vi "PH_Sequencer_Watch.ProcEvents.vi"(0 "i ref in":refnum<vi>, 5 "error in (no error)":errorcluster) -> (14 "i ref out":refnum<vi>, 19 "error out":errorcluster)   [LabVIEW 2014, in "PH_Sequencer_Watch.lvlib"]
doc: "This method is used to define the events the object will listen to. Add your own events here."
uses:
  PH_Sequencer_Watch.lvlib
  PH_Beckhoff_PP_PU/PH_Beckhoff_PP_PU.HV Meas Tags.ctl
  PH_PP_Common/PH_PP_Common.PSU Tags.ctl
  PH_Common/DIM/PH_DIM.Event Declarer.ctl
  PH_PowerUnit_BaseClass/PH_PowerUnit_BaseClass.PP PU Tags.ctl
  CSCore/BaseProcess/BaseProcess.lvlib
  PH_Common/PH_Common.lvlib
  PH_Beckhoff_PP_PU/PH_Beckhoff_PP_PU.lvlib
  PH_PowerUnit_BaseClass/PH_PowerUnit_BaseClass.lvlib
  PH_PP_Common/PH_PP_Common.lvlib
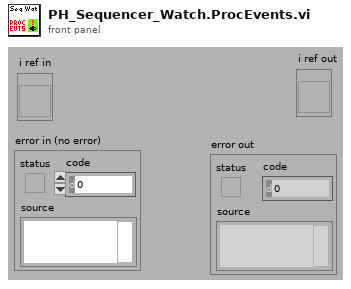
[diagram p1: front panel]
types:
  T1 = typedef "PH_PP_Common.lvlib/PH_PP_Common.PSU Tags.ctl" = enum16{"voltage-indicator", "peak-detect", "current", "voltage", "inihibit-indicator", "end-of-charge", "HV-on-indicator", "overtemperature", "interlock-indicator", "load-fault", "sum-fault", "HV-off-indicator", "DC-ok", "inhibit", "HV-on", "interlock", "reset", "Status", "Limits"}
  T2 = typedef "PH_Beckhoff_PP_PU.lvlib/PH_Beckhoff_PP_PU.HV Meas Tags.ctl" = enum16{"voltage-raw", "voltage"}
  T3 = typedef "PH_Common.lvlib/PH_DIM.Event Declarer.ctl" = cluster{"Service Name":string, "Selector":string}
  T4 = typedef "PH_PowerUnit_BaseClass.lvlib/PH_PowerUnit_BaseClass.PP PU Tags.ctl" = enum16{"Waiting-Time", "PU-in-Use"}
  T5 = typedef "PH_Sequencer_Watch.lvlib/PH_Sequencer_Watch.i attribute.ctl" = cluster{"GUI Refs":cluster{"Shot ID":refnum<vi>, "Sequencer SM State":refnum<vi>, "Remaining Time":refnum<vi>, "PHELIX_Timing_T2":refnum<vi>, "T2-Unit-Dummy":refnum<vi>, "fs_Synchrolock_Watch":refnum<vi>, "Experiment_Vacuum_Control_Experiment":refnum<vi>}, "Status Synchrolock":T6, "Exp - Pressure":dbl, "Exp - Limit":dbl, "Heads":T7[], "Refs BooleanState":refnum<vi>[]}
  T6 = typedef "PH_StatusHandler.lvlib/PH_StatusHandler.Status.ctl" = i16
  T7 = typedef "PH_Sequencer_Watch.lvlib/PH_Sequencer_Watch.Head Information.ctl" = cluster{"Ref Volt":refnum<vi>, "PU":T8}
  T8 = typedef "PH_PP_Common.lvlib/PH_PP_Common.PUs.ctl" = enum16{"no Info", "PA-19mm-1", "PA-19mm-2", "PA-45mm-PILC", "PA-45mm-MAIN", "MA-PU-1", "MA-PU-2", "MA-PU-3", "MA-PU-4", "MA-PU-5", "MA-PU-6", "MA-FR", "MA-PILC", "PA-45mm-DP"}
  T9 = typedef "PH_PP_Common.lvlib/PH_PP_Common.PSU Type.ctl" = enum16{"none", "Maxwell Standard", "DEL", "Maxwell ALE", "Continuum 601k"}
  T10 = typedef "BaseProcess.lvlib/BaseProcess.event definition.ctl" = cluster{"CAEEvtDef":T11, "Data Descriptor":T12}
  T11 = typedef "CAEObj.lvlib/CAEObj.event definition.ctl" = cluster{"URL":string, "enable":bool, "ignoreResID":bool}
  T12 = typedef "BaseProcess.lvlib/BaseProcess.descriptor string definition.ctl" = string
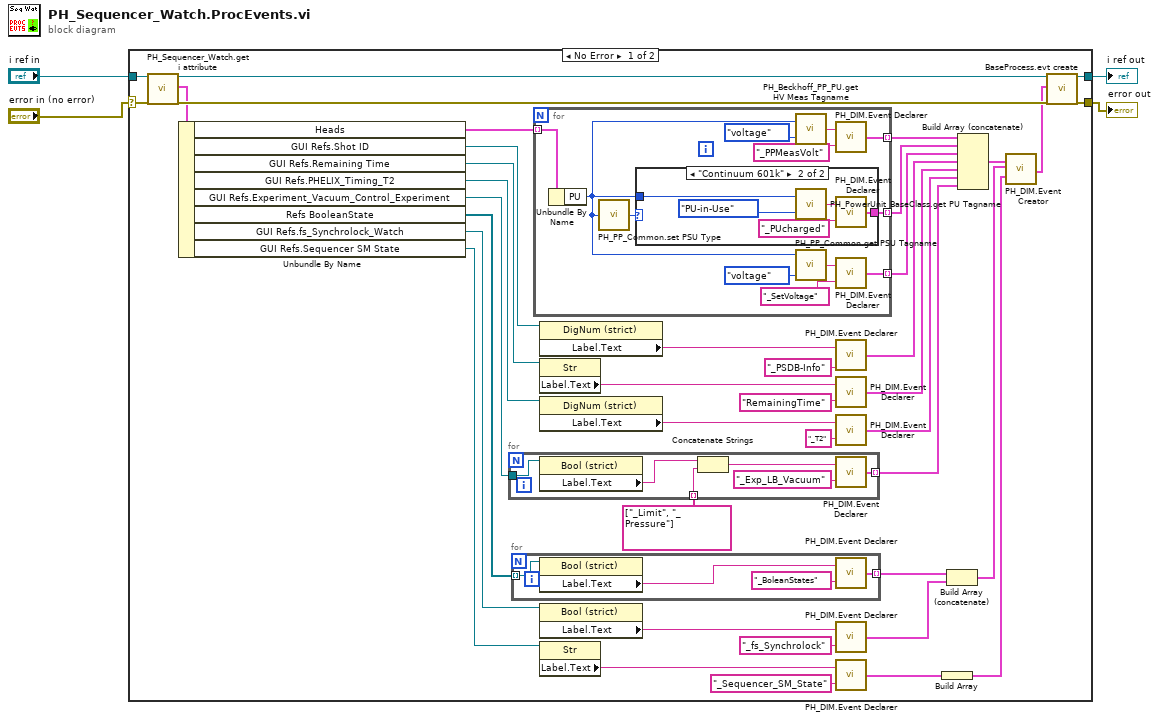
[diagram p0: block diagram]
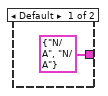
[diagram p2: hidden frame]
diagram:
  n1 = case shown="No Error" "error in (no error)" {
    selector: "error in (no error)" -> [w39 w73]
    tunnel: "i ref in" -> [w42 w74]
    tunnel: [w41 w74] -> w3
    tunnel: [w40 w73] -> w2
    frame No Error {
      n2 = call "PH_Sequencer_Watch.get i attribute.vi"("i ref in"=w42, "error in (no error)"=w39) -> ("i ref out"=w44:refnum<vi>, "i attribute"=w36:T5, "error out"=w43:errorcluster)  [unwired: 15 in]
      n3 = Unbundle By Name(w36) -> ("Heads"=w25:T7[], "GUI Refs.Shot ID"=w30:refnum<vi>, "GUI Refs.Remaining Time"=w32:refnum<vi>, "GUI Refs.PHELIX_Timing_T2"=w20:refnum<vi>, "GUI Refs.Experiment_Vacuum_Control_Experiment"=w10:refnum<vi>, "Refs BooleanState"=w17:refnum<vi>[], "GUI Refs.fs_Synchrolock_Watch"=w14:refnum<vi>, "GUI Refs.Sequencer SM State"=w7:refnum<vi>)
      n4 = for {
        tunnel: [w49] -> w8 mode=indexing
        tunnel: w10 -> [w47]
        tunnel: string[] ["_Limit", "_Pressure"] -> [w45] mode=indexing
        n5 = property class="Bool (strict)"(reference=w47) -> ("Label.Text"=w48:string)  [unwired: 1 in, 2 out]
        n6 = Concatenate Strings(w48, w45) -> (w46:string)
        n7 = call "PH_DIM.Event Declarer.vi"("Selector"="_Exp_LB_Vacuum" ("URL"), "Service Name"=w46) -> ("declared DIM Event"=w49:T3)
      }
      n8 = for {
        tunnel: [w53] -> w15 mode=indexing
        tunnel: w17 -> [w51] mode=indexing
        n9 = property class="Bool (strict)"(reference=w51) -> ("Label.Text"=w52:string)  [unwired: 1 in, 2 out]
        n10 = call "PH_DIM.Event Declarer.vi"("Selector"="_BoleanStates" ("URL"), "Service Name"=w52) -> ("declared DIM Event"=w53:T3)
      }
      n11 = for {
        tunnel: w25 -> [w64] mode=indexing
        tunnel: [w65] -> w23 mode=indexing
        tunnel: [w61] -> w6 mode=indexing
        tunnel: [w55] -> w5 mode=indexing
        n12 = Unbundle By Name(w64) -> ("PU"=w59:T8)
        n13 = call "PH_PP_Common.set PSU Type.vi"("PU"=w59) -> ("PSU Type"=w60:T9)
        n14 = case shown="\"Continuum 601k\"" w60 {
          tunnel: w59 -> [_ w71]
          tunnel: [T3 {"Service Name"="N/A", "Selector"="N/A"} ("declared DIM Event") w70] -> w61
          frame Default {
          }
          frame "Continuum 601k" {
            n15 = call "PH_PowerUnit_BaseClass.get PU Tagname.vi"("PU Tag"=PH_PowerUnit_BaseClass.PP_PU_Tags."PU-in-Use", "PU"=w71) -> ("PU Tagname"=w72:string)
            n16 = call "PH_DIM.Event Declarer.vi"("Selector"="_PUcharged", "Service Name"=w72) -> ("declared DIM Event"=w70:T3)
          }
        }
        n17 = call "PH_Beckhoff_PP_PU.get HV Meas Tagname.vi"("HV Meas Tag"=PH_Beckhoff_PP_PU.HV_Meas_Tags."voltage", "PU"=w59) -> ("HV Meas Tagname"=w63:string)
        n18 = call "PH_PP_Common.get PSU Tagname.vi"("PSU Tag"=PH_PP_Common.PSU_Tags."voltage", "PU"=w59) -> ("PSU Tagname"=w57:string)  [unwired: 1 in]
        n19 = call "PH_DIM.Event Declarer.vi"("Selector"="_PPMeasVolt" ("URL"), "Service Name"=w63) -> ("declared DIM Event"=w65:T3)
        n20 = call "PH_DIM.Event Declarer.vi"("Selector"="_SetVoltage", "Service Name"=w57) -> ("declared DIM Event"=w55:T3)
      }
      n21 = property class="DigNum (strict)"(reference=w30) -> ("Label.Text"=w29:string)  [unwired: 1 in, 2 out]
      n22 = property class="Str"(reference=w32) -> ("Label.Text"=w26:string)  [unwired: 1 in, 2 out]
      n23 = property class="DigNum (strict)"(reference=w20) -> ("Label.Text"=w19:string)  [unwired: 1 in, 2 out]
      n24 = property class="Bool (strict)"(reference=w14) -> ("Label.Text"=w13:string)  [unwired: 1 in, 2 out]
      n25 = property class="Str"(reference=w7) -> ("Label.Text"=w28:string)  [unwired: 1 in, 2 out]
      n26 = call "PH_DIM.Event Declarer.vi"("Selector"="_PSDB-Info" ("URL"), "Service Name"=w29) -> ("declared DIM Event"=w37:T3)
      n27 = call "PH_DIM.Event Declarer.vi"("Selector"="RemainingTime" ("URL"), "Service Name"=w26) -> ("declared DIM Event"=w31:T3)
      n28 = call "PH_DIM.Event Declarer.vi"("Selector"="_T2", "Service Name"=w19) -> ("declared DIM Event"=w18:T3)
      n29 = call "PH_DIM.Event Declarer.vi"("Selector"="_fs_Synchrolock", "Service Name"=w13) -> ("declared DIM Event"=w12:T3)
      n30 = call "PH_DIM.Event Declarer.vi"("Selector"="_Sequencer_SM_State", "Service Name"=w28) -> ("declared DIM Event"=w34:T3)
      n31 = Build Array(w34) -> (w24:T3[])
      n32 = Build Array (concatenate)(w15, w12) -> (w16:T3[])
      n33 = Build Array (concatenate)(w23, w6, w5, w37, w31, w18, w8) -> (w38:T3[])
      n34 = call "PH_DIM.Event Creator.vi"("Trendmessage Services"=w38, "Status Services"=w16, "SM State Services"=w24) -> ("DIM Service Events"=w22:T10[])  [unwired: 16 in]
      n35 = call "BaseProcess.evt create.vi"("i ref in"=w44, "newEvents"=w22, "error in (no error)"=w43) -> ("i ref out"=w41:refnum<vi>, "error out"=w40:errorcluster)  [unwired: 13 in, 2 out]
    }
    frame Error {
    }
  }
  "i ref out" <- w3
  "error out" <- w2
